vi "Finished Late.vi"(8 "error in (no error)":errorcluster, 11 "Finished \nLate?":bool) -> (0 "error out":errorcluster, 2 "# Finished\nLate counter":dbl, 3 "Finished \nLate?":bool)   [LabVIEW 2018, in "Timing.lvlib"]
doc: "Increments a counter each time loop finishes late"
uses:
  Timing.lvlib
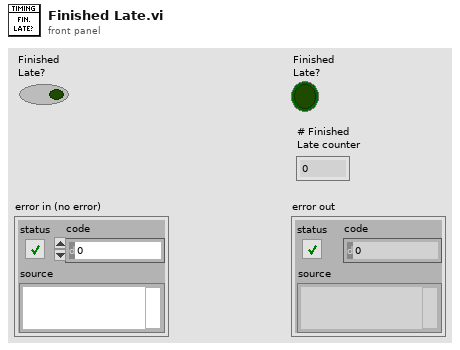
[diagram p1: front panel]
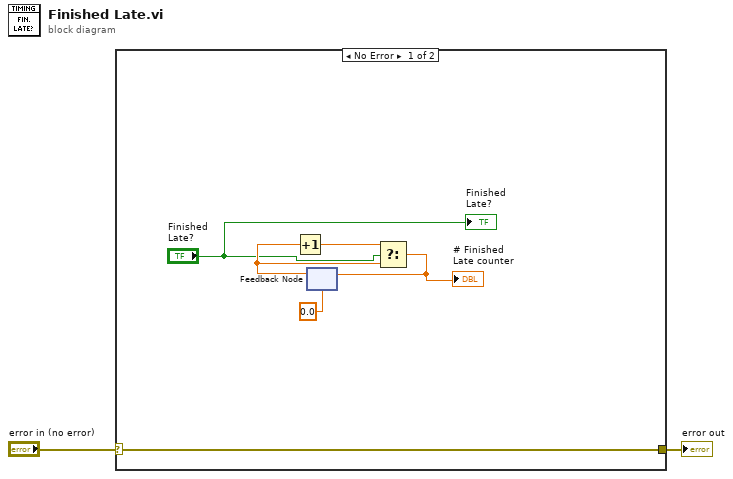
[diagram p0: block diagram]
diagram:
  n1 = case shown="No Error" "error in (no error)" {
    selector: "error in (no error)" -> [w3 w9]
    tunnel: [w3 w9] -> w1
    frame No Error {
      n2 = feedback #1(0.0) -> (w7:dbl)
      n3 = Increment(x=w7) -> (x+1=w8:dbl)
      n4 = Select(t=w8, s="Finished \nLate?", f=w7) -> (s? t:f=w5:dbl)
      "# Finished\nLate counter" <- w5
      n5 = feedback-in #1 ("2")(w5) -> ()
      "Finished \nLate?" <- "Finished \nLate?"
    }
    frame Error {
    }
  }
  "error out" <- w1
